vi "Misc Ignore Timeout Error.vi"(8 "error in (no error)":errorcluster) -> (0 "error out":errorcluster, 2 "timed out?":bool)   [LabVIEW 2011, in "Misc VIs.lvlib"]
uses:
  Misc VIs.lvlib
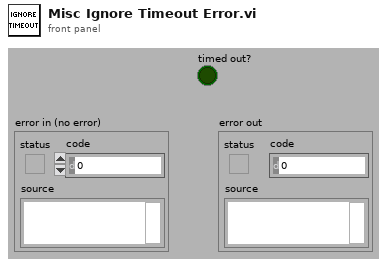
[diagram p1: front panel]
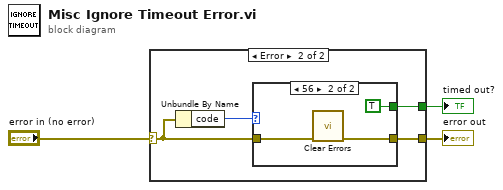
[diagram p0: block diagram]
diagram:
  n1 = case shown="Error" "error in (no error)" {
    selector: "error in (no error)" -> [w4 w7]
    tunnel: [w4 w6] -> w2
    tunnel: [_ w5] -> w1
    frame No Error {
    }
    frame Error {
      n2 = Unbundle By Name(w7) -> ("code"=w8:i32)
      n3 = case shown="56" w8 {
        tunnel: w7 -> [w9 w12]
        tunnel: [w9 w11] -> w6
        tunnel: [_ TRUE] -> w5
        frame 0, Default {
        }
        frame 56 {
          n4 = call <vilib>:"Clear Errors.vi"("error in (no error)"=w12) -> ("error out"=w11:errorcluster)  [unwired: 6 out]
        }
      }
    }
  }
  "error out" <- w2
  "timed out?" <- w1
